vi "Get Name.vi"(8 "error in (no error)":errorcluster, 11 "Orange Plugin in":refnum<class "Orange Plugin.lvclass">) -> (0 "error out":errorcluster, 2 "Get Name":string, 3 "Orange Plugin out":refnum<class "Orange Plugin.lvclass">)   [LabVIEW 2011, in "Orange Plugin.lvclass"]
uses:
  Orange Plugin.lvclass
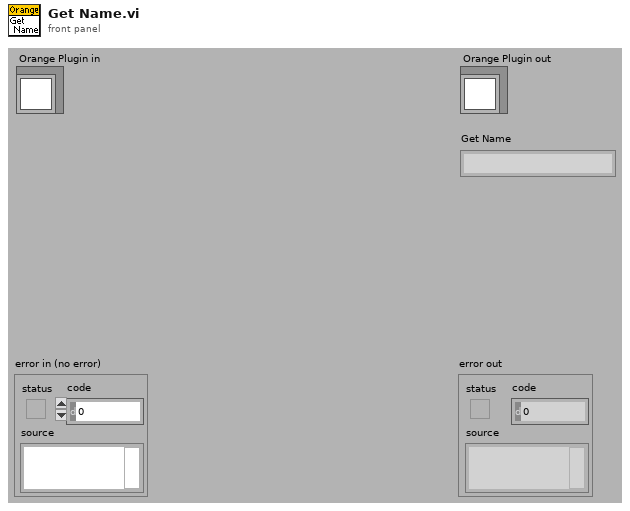
[diagram p1: front panel]
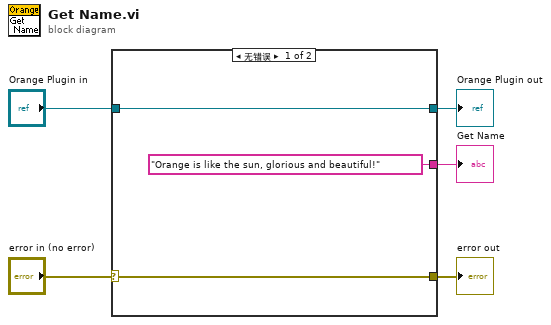
[diagram p0: block diagram]
diagram:
  n1 = case shown="无错误" "error in (no error)" {
    selector: "error in (no error)" -> [w8 w10]
    tunnel: [w8 w10] -> w4
    tunnel: ["Orange is like the sun, glorious and beautiful!" _] -> w3
    tunnel: [w6 w9] -> w2
    tunnel: "Orange Plugin in" -> [w6 w9]
    frame No Error {
    }
    frame Error {
    }
  }
  "error out" <- w4
  "Get Name" <- w3
  "Orange Plugin out" <- w2
